vi "OFDM-A1信道估计.vi"(1 "信道1导频输入":cdb[](array[numeric])) -> (0 "输出":cdb[](array[numeric]))   [LabVIEW 2018]
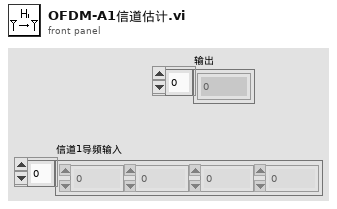
[diagram p1: front panel]
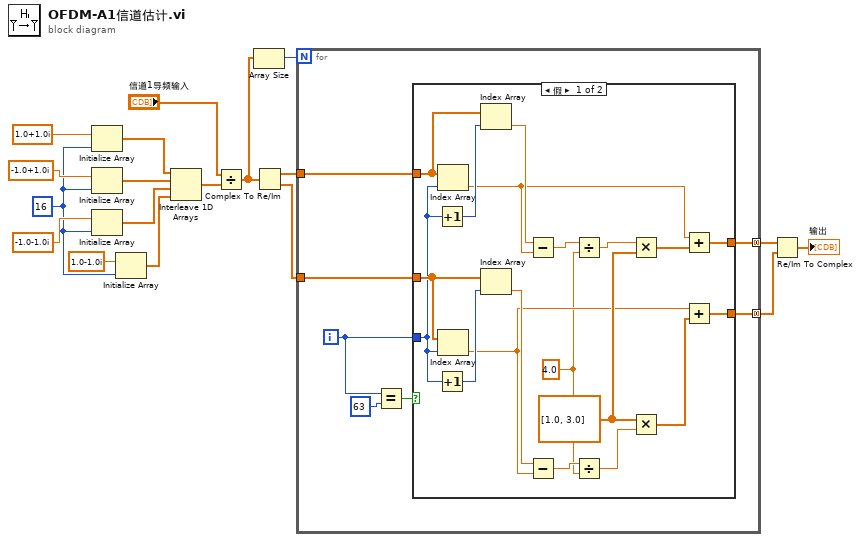
[diagram p0: block diagram]
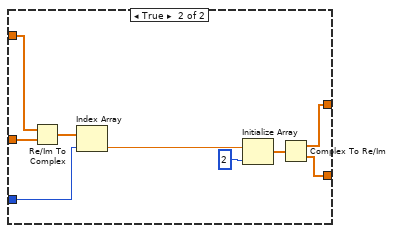
[diagram p2: hidden frame]
diagram:
  w2 = 16
  n1 = Initialize Array(cdb 1.0+1.0i, w2) -> (w9:cdb[])
  n2 = Initialize Array(cdb -1.0+1.0i, w2) -> (w6:cdb[])
  n3 = Initialize Array(cdb -1.0-1.0i, w2) -> (w7:cdb[])
  n4 = Initialize Array(cdb 1.0-1.0i, w2) -> (w8:cdb[])
  n5 = Interleave 1D Arrays(w9, w6, w7, w8) -> (w1:cdb[])
  n6 = Divide(x="信道1导频输入", y=w1) -> (x/y=w18:cdb[])
  n7 = Array Size(array=w18) -> (size(s)=w17:i32)
  n8 = Complex To Re/Im(x + iy=w18) -> (x=w16:dbl[], y=w15:dbl[])
  n9 = for {
    N: w17 -> [_]
    tunnel: w16 -> [w23]
    tunnel: w15 -> [w21]
    tunnel: [w20] -> w14 mode=concatenating
    tunnel: [w19] -> w13 mode=concatenating
    i -> [w22]
    n10 = Equal?(x=w22, y=63) -> (x = y?=w24:bool)
    n11 = case shown="假" w24 {
      tunnel: w23 -> [w44 w53]
      tunnel: w22 -> [w41 w50]
      tunnel: w21 -> [w42 w52]
      tunnel: [w28 w47] -> w20
      tunnel: [w27 w46] -> w19
      frame False {
        w26 = 4.0 ("y")
        w31 = dbl[] [1.0, 3.0] ("y")
        n12 = Increment(x=w41) -> (x+1=w43:i32)
        n13 = Increment(x=w41) -> (x+1=w40:i32)
        n14 = Index Array(array=w44, index=w41) -> (element=w35:dbl)
        n15 = Index Array(array=w42, index=w41) -> (element=w30:dbl)
        n16 = Index Array(array=w44, index=w43) -> (element=w39:dbl)
        n17 = Index Array(array=w42, index=w40) -> (element=w34:dbl)
        n18 = Subtract(x=w39, y=w35) -> (x-y=w38:dbl)
        n19 = Subtract(x=w34, y=w30) -> (x-y=w33:dbl)
        n20 = Divide(x=w38, y=w26) -> (x/y=w37:dbl)
        n21 = Divide(x=w33, y=w26) -> (x/y=w32:dbl)
        n22 = Multiply(x=w37, y=w31) -> (x*y=w36:dbl[])
        n23 = Multiply(x=w31, y=w32) -> (x*y=w29:dbl[])
        n24 = Add(x=w35, y=w36) -> (x+y=w28:dbl[])
        n25 = Add(x=w30, y=w29) -> (x+y=w27:dbl[])
      }
      frame True {
        n26 = Re/Im To Complex(1:w52, 2:w53) -> (0:w51:cdb[])
        n27 = Index Array(array=w51, index=w50) -> (element=w49:cdb)
        n28 = Initialize Array(w49, 2 ("维数大小")) -> (w48:cdb[])
        n29 = Complex To Re/Im(x + iy=w48) -> (x=w47:dbl[], y=w46:dbl[])
      }
    }
  }
  n30 = Re/Im To Complex(1:w13, 2:w14) -> (0:→"输出":cdb[])
